vi "uArm_SelectGCode.vi"(7 "Gripper Closed":bool, 8 "error in (no error)":errorcluster, 9 "rightTrig":dbl, 10 "full read buffer in":string, 11 "VISA Refnum in":refnum<visa-resource-name>) -> (0 "error out":errorcluster, 1 "Command":string, 2 "full read buffer out":string, 3 "VISA Refnum out":refnum<visa-resource-name>)   [LabVIEW 2017]
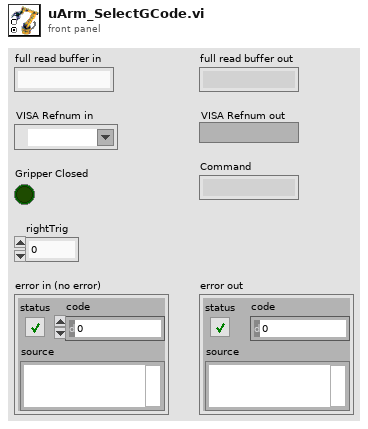
[diagram p1: front panel]
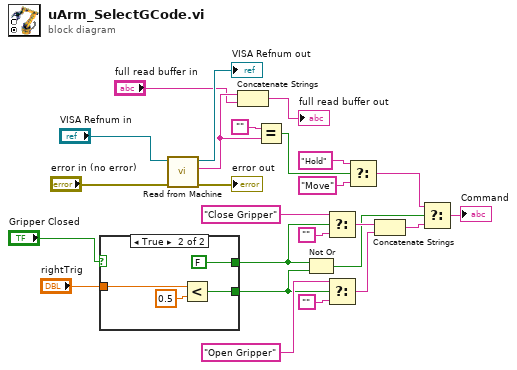
[diagram p0: block diagram]
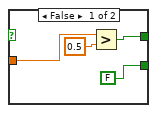
[diagram p2: hidden frame]
diagram:
  n1 = case shown="True" "Gripper Closed" {
    tunnel: "rightTrig" -> [w29 w33]
    tunnel: [FALSE w31] -> w6
    tunnel: [w27 FALSE] -> w17
    frame False {
      n2 = Greater?(x=w29, y=0.5) -> (0:w27:bool)
    }
    frame True {
      n3 = Less?(x=w33, y=0.5) -> (x < y?=w31:bool)
    }
  }
  n4 = call "Read from Machine.vi"("error in (no error)"="error in (no error)", "Machine In"="VISA Refnum in") -> ("error out"=→"error out":errorcluster, "read buffer"=w10:string, "Machine Out"=→"VISA Refnum out":refnum<visa-resource-name>)  [unwired: 7 in]
  n5 = Concatenate Strings(w10, "full read buffer in") -> (→"full read buffer out":string)
  n6 = Equal?(x="", y=w10) -> (x = y?=w12:bool)
  n7 = Not Or(1:w6, 2:w17) -> (0:w7:bool)
  n8 = Select(t="Close Gripper", s=w17, f="") -> (s? t:f=w15:string)
  n9 = Select(t="Open Gripper", s=w6, f="") -> (s? t:f=w16:string)
  n10 = Select(t="Hold", s=w12, f="Move") -> (s? t:f=w23:string)
  n11 = Concatenate Strings(w15, w16) -> (w24:string)
  n12 = Select(t=w23, s=w7, f=w24) -> (s? t:f=→"Command":string)
